vi "getInheritanceChain.vi"(8 "error in (no error)":errorcluster, 11 "PriorityNode in":refnum<class "PriorityNode.lvclass">) -> (0 "error out":errorcluster, 2 "Inheritance Chain":string[](array[string]), 3 "PriorityNode out":refnum<class "PriorityNode.lvclass">)   [LabVIEW 2009, in "PriorityNode.lvclass"]
doc: "Returns the inheritance chain."
uses:
  PriorityNode.lvclass
  LLNode/LLNode.lvclass
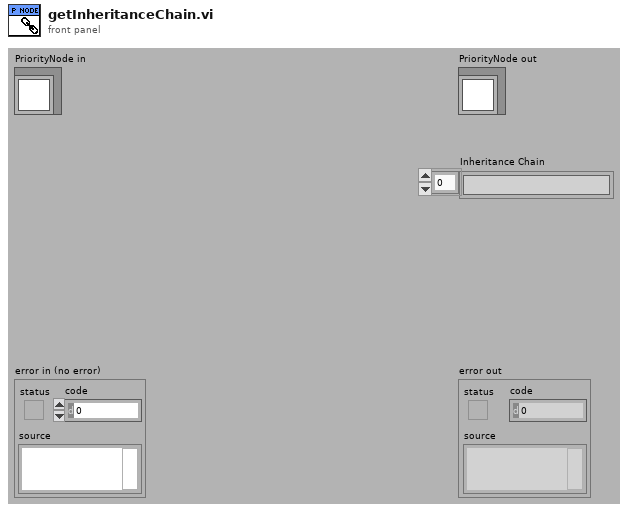
[diagram p1: front panel]
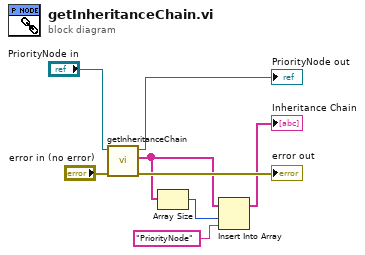
[diagram p0: block diagram]
diagram:
  n1 = call-parent "getInheritanceChain.vi"("error in (no error)"="error in (no error)", "LLNode in"="PriorityNode in") -> ("error out"=→"error out":errorcluster, "Inheritance Chain"=w4:string[], "LLNode out"=→"PriorityNode out":refnum<class "PriorityNode.lvclass">)  [unwired: 7 in]
  n2 = Array Size(array=w4) -> (size(s)=w3:i32)
  n3 = Insert Into Array(array=w4, index=w3, new element="PriorityNode" ("new element/subarray")) -> (→"Inheritance Chain":string[])
